vi "S2C_M2p5942_Poly_TestBed.vi"() -> ()   [LabVIEW 2015]
uses:
  S2C_M2p5942_Poly_Initialize.vi
  S2C_M2p5942_Poly_Channels.vi
  S2C_M2p5942_Poly_ClockSettings.vi
  S2C_M2p5942_Poly_ModeSettings.vi
  S2C_M2p5942_Poly_MultiPurposeIO.vi
  S2C_M2p5942_Poly_TriggerSettings.vi
  S2C_M2p5942_Poly_Acquisition.vi
panel:
  out "Error Out":errorcluster
  in  "Error In":errorcluster
  out "Response":T1
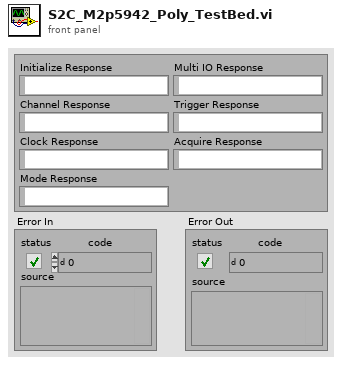
[diagram p1: front panel]
types:
  T1 = cluster{"Initialize Response":string, "Channel Response":string, "Clock Response":string, "Mode Response":string, "Multi IO Response":string, "Trigger Response":string, "Acquire Response":string}
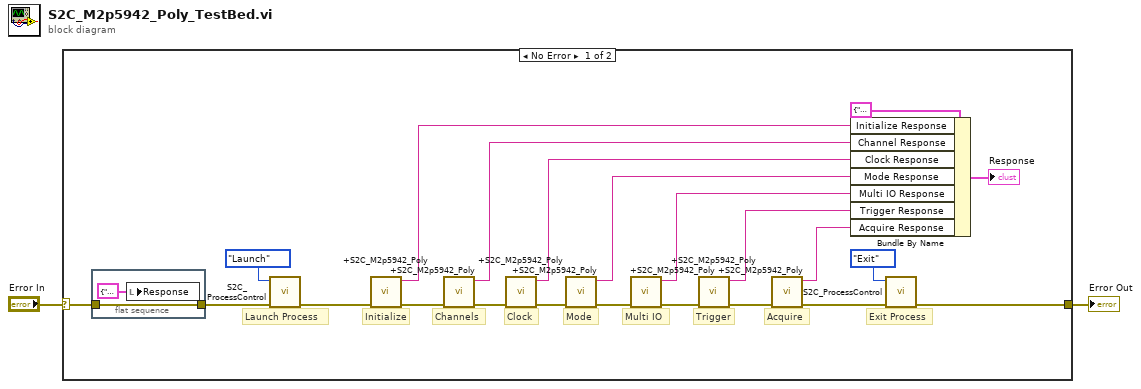
[diagram p0: block diagram]
diagram:
  n1 = case shown="No Error" "Error In" {
    selector: "Error In" -> [w21 w27]
    tunnel: [w22 w27] -> w1
    frame No Error {
      # "Acquire"
      # "Trigger"
      # "Multi IO"
      # "Mode"
      # "Clock"
      # "Channels"
      # "Initialize"
      # "Exit Process"
      # "Launch Process"
      n2 = flat-sequence {
        tunnel: w21 -> [w26]
        tunnel: [w26] -> w20
        frame #0 {
          n3 = local write "Response"(T1 {"Initialize Response"="", "Channel Response"="", "Clock Response"="", "Mode Response"="", "Multi IO Response"="", "Trigger Response"="", "Acquire Response"=""} ("Response")) -> ()
        }
      }
      n4 = call "S2C_ProcessControl.vi"("Error In"=w20, "Action"=enum16{"Launch", "Exit"}."Launch") -> ("Error Out"=w19:errorcluster)  [unwired: 9 in]
      n5 = call-poly "+S2C_M2p5942_Poly.vi"("Error In"=w19) -> ("Error Out"=w18:errorcluster, "Response"=w12:string)  [unwired: 9 in]
      n6 = call-poly "+S2C_M2p5942_Poly.vi"("Error In"=w18) -> ("Error Out"=w17:errorcluster, "Response"=w11:string)  [unwired: 9 in]
      n7 = call-poly "+S2C_M2p5942_Poly.vi"("Error In"=w17) -> ("Error Out"=w6:errorcluster, "Response"=w10:string)  [unwired: 9 in]
      n8 = call-poly "+S2C_M2p5942_Poly.vi"("Error In"=w6) -> ("Error Out"=w5:errorcluster, "Response"=w9:string)  [unwired: 9 in]
      n9 = call-poly "+S2C_M2p5942_Poly.vi"("Error In"=w5) -> ("Error Out"=w4:errorcluster, "Response"=w8:string)  [unwired: 9 in]
      n10 = call-poly "+S2C_M2p5942_Poly.vi"("Error In"=w4) -> ("Error Out"=w3:errorcluster, "Response"=w7:string)  [unwired: 9 in]
      n11 = call-poly "+S2C_M2p5942_Poly.vi"("Error In"=w3) -> ("Error Out"=w16:errorcluster, "Response"=w13:string)  [unwired: 9 in]
      n12 = Bundle By Name(cluster=T1 {"Initialize Response"="", "Channel Response"="", "Clock Response"="", "Mode Response"="", "Multi IO Response"="", "Trigger Response"="", "Acquire Response"=""} ("Response"), "Initialize Response"=w12, "Channel Response"=w11, "Clock Response"=w10, "Mode Response"=w9, "Multi IO Response"=w8, "Trigger Response"=w7, "Acquire Response"=w13) -> (→"Response":T1)
      n13 = call "S2C_ProcessControl.vi"("Error In"=w16, "Action"=enum16{"Launch", "Exit"}."Exit") -> ("Error Out"=w22:errorcluster)  [unwired: 9 in]
    }
    frame Error {
    }
  }
  "Error Out" <- w1
